vi "Keyboard.vi"(8 "Error In":errorcluster, 9 "Enable (F)":bool, 11 "VISA resource name":refnum<visa-resource-name>) -> (0 "Error Out":errorcluster, 3 "dup VISA resource name":refnum<visa-resource-name>)   [LabVIEW 2011, in "MGC647C.lvlib"]
doc: "Enable/disable keyboard."
uses:
  <instrlib>/MGC647C/MGC647C.lvlib
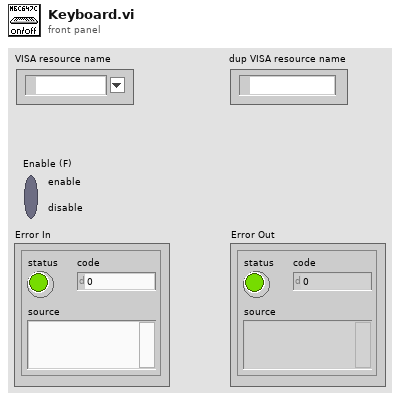
[diagram p1: front panel]
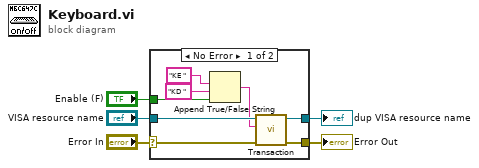
[diagram p0: block diagram]
diagram:
  n1 = case shown="No Error" "Error In" {
    selector: "Error In" -> [w10 w15]
    tunnel: "VISA resource name" -> [w13 w14]
    tunnel: [w12 w14] -> w4
    tunnel: [w11 w15] -> w3
    tunnel: "Enable (F)" -> [w9 _]
    frame No Error {
      n2 = Append True/False String(1:w9, 2:"KD " ("string (\"\")"), 3:"KE " ("string (\"\")")) -> (0:w6:string)  [unwired: 1 in]
      n3 = call <instrlib>:"Transaction.vi"("Error In"=w10, "Command"=w6, "VISA resource name"=w13) -> ("Error Out"=w11:errorcluster, "dup VISA resource name"=w12:refnum<visa-resource-name>)  [unwired: 6 in, 1 out]
    }
    frame Error {
    }
  }
  "dup VISA resource name" <- w4
  "Error Out" <- w3
